vi "set_lc_end.vi"(8 "yw":string, 9 "state":string, 11 "lc_num":string) -> (2 "error":errorcluster)   [LabVIEW 2017, in "Lib_code.lvlib"]
uses:
  Lib_code.lvlib
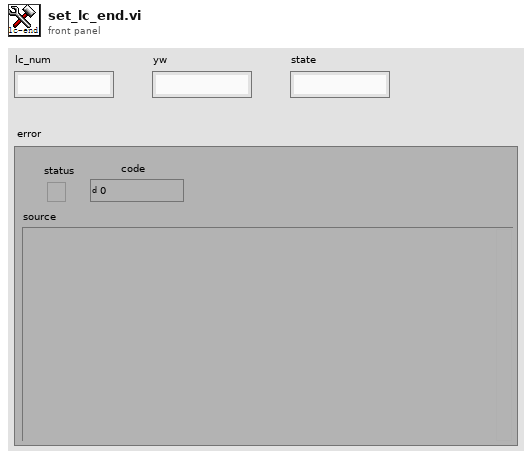
[diagram p1: front panel]
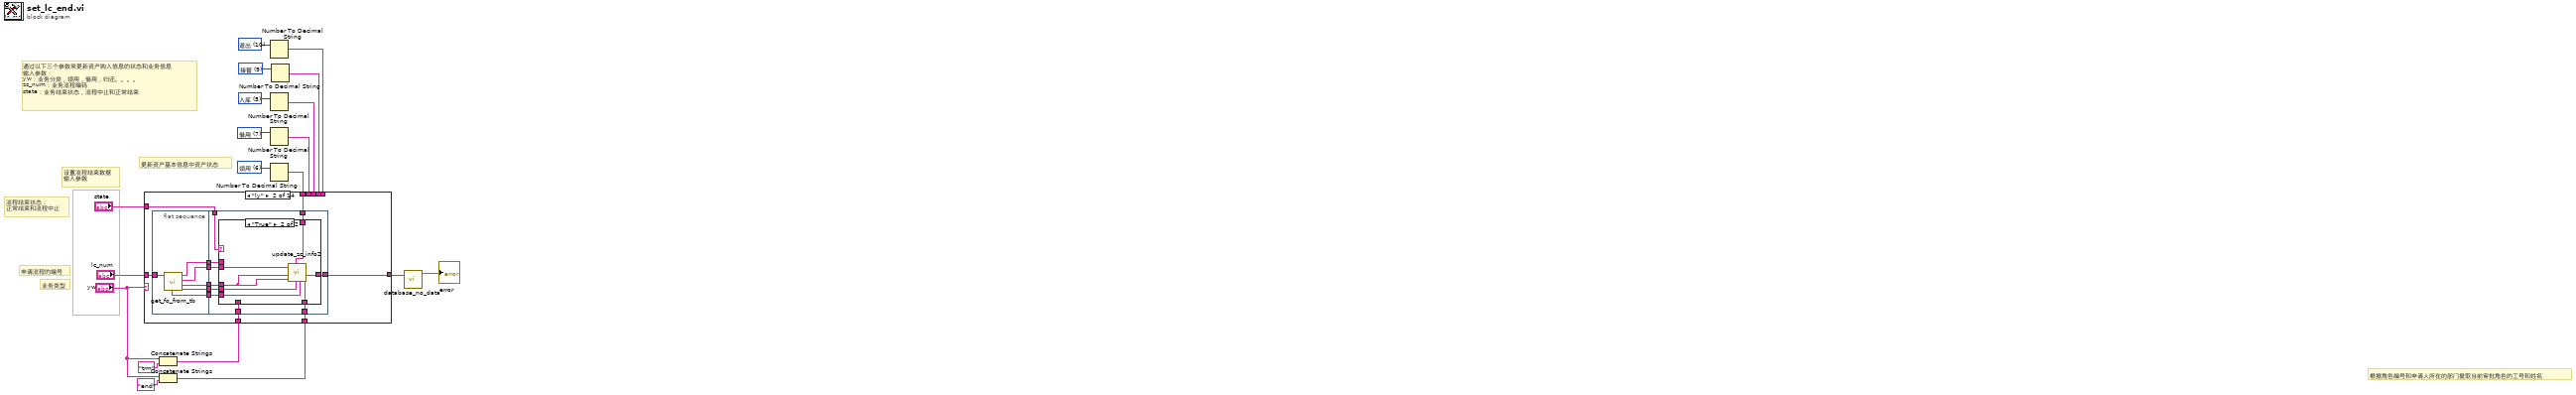
[diagram p0: block diagram]
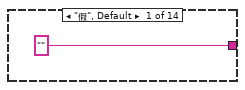
[diagram p2: hidden frame]
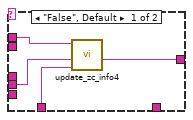
[diagram p3: hidden frame]
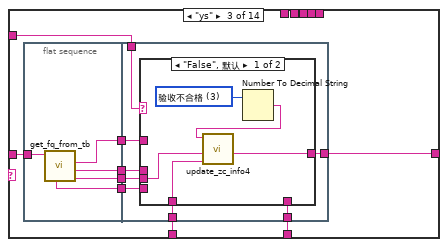
[diagram p4: hidden frame]
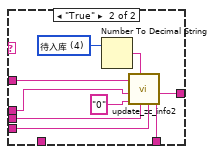
[diagram p5: hidden frame]
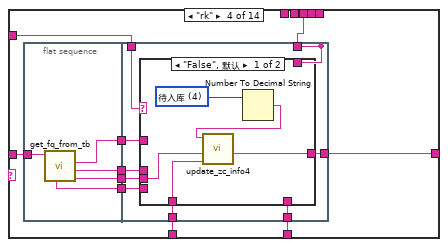
[diagram p6: hidden frame]
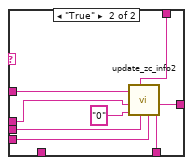
[diagram p7: hidden frame]
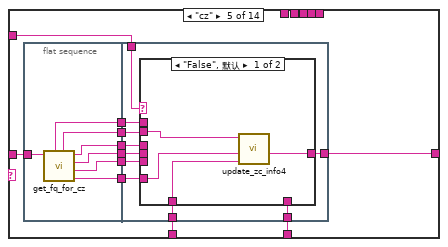
[diagram p8: hidden frame]
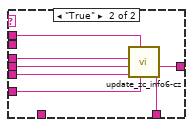
[diagram p9: hidden frame]
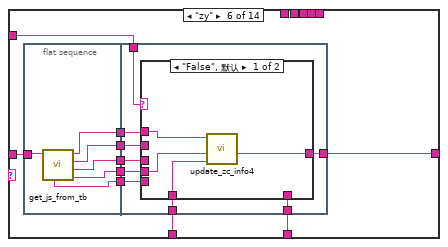
[diagram p10: hidden frame]
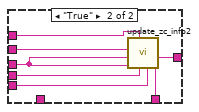
[diagram p11: hidden frame]
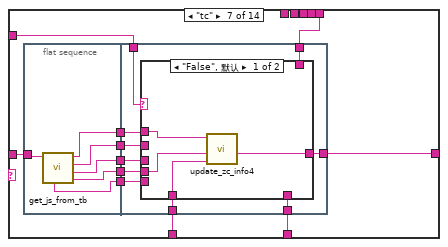
[diagram p12: hidden frame]
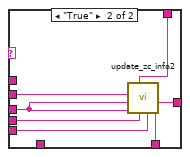
[diagram p13: hidden frame]
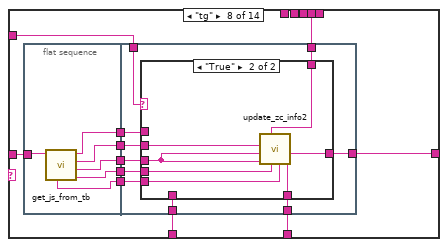
[diagram p14: hidden frame]
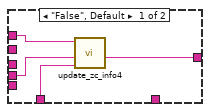
[diagram p15: hidden frame]
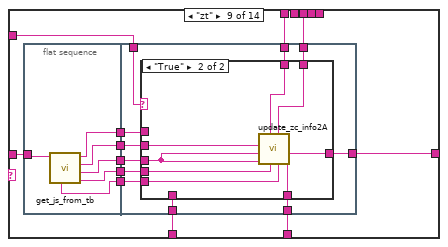
[diagram p16: hidden frame]
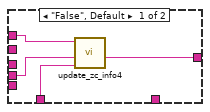
[diagram p17: hidden frame]
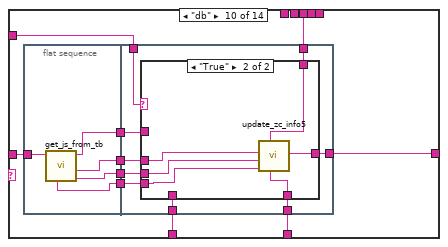
[diagram p18: hidden frame]
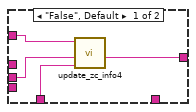
[diagram p19: hidden frame]
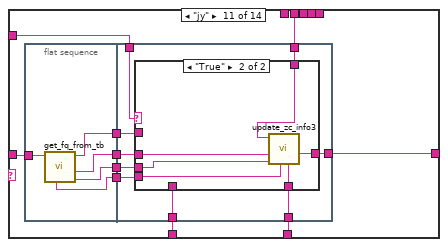
[diagram p20: hidden frame]
diagram:
  w2 = u8 10 items=["待验收"=1, "无需验收"=2, "验收不合格"=3, "待入库"=4, "入库"=5, "领用"=6, "借用"=7, "托管"=8, "接管"=9, "退出"=10, "出库在用"=11, "盘亏"=12, "出售"=13, "报废"=14, "领用中"=120, "退库中"=121, "借用中"=122, "归还中"=123, "转移中"=124, "调拨中"=125, "借调中"=126, "托管中"=127, "终止托管中"=128, "退出中"=129, "处置中"=130] ("借用状态")
  w5 = u8 6 items=["待验收"=1, "无需验收"=2, "验收不合格"=3, "待入库"=4, "入库"=5, "领用"=6, "借用"=7, "托管"=8, "接管"=9, "退出"=10, "出库在用"=11, "盘亏"=12, "出售"=13, "报废"=14, "领用中"=120, "退库中"=121, "借用中"=122, "归还中"=123, "转移中"=124, "调拨中"=125, "借调中"=126, "托管中"=127, "终止托管中"=128, "退出中"=129, "处置中"=130] ("借用状态")
  w6 = u8 7 items=["待验收"=1, "无需验收"=2, "验收不合格"=3, "待入库"=4, "入库"=5, "领用"=6, "借用"=7, "托管"=8, "接管"=9, "退出"=10, "出库在用"=11, "盘亏"=12, "出售"=13, "报废"=14, "领用中"=120, "退库中"=121, "借用中"=122, "归还中"=123, "转移中"=124, "调拨中"=125, "借调中"=126, "托管中"=127, "终止托管中"=128, "退出中"=129, "处置中"=130] ("借用状态")
  w7 = u8 5 items=["待验收"=1, "无需验收"=2, "验收不合格"=3, "待入库"=4, "入库"=5, "领用"=6, "借用"=7, "托管"=8, "接管"=9, "退出"=10, "出库在用"=11, "盘亏"=12, "出售"=13, "报废"=14, "领用中"=120, "退库中"=121, "借用中"=122, "归还中"=123, "转移中"=124, "调拨中"=125, "借调中"=126, "托管中"=127, "终止托管中"=128, "退出中"=129, "处置中"=130] ("借用状态")
  w4 = u8 9 items=["待验收"=1, "无需验收"=2, "验收不合格"=3, "待入库"=4, "入库"=5, "领用"=6, "借用"=7, "托管"=8, "接管"=9, "退出"=10, "出库在用"=11, "盘亏"=12, "出售"=13, "报废"=14, "领用中"=120, "退库中"=121, "借用中"=122, "归还中"=123, "转移中"=124, "调拨中"=125, "借调中"=126, "托管中"=127, "终止托管中"=128, "退出中"=129, "处置中"=130] ("借用状态")
  # "更新资产基本信息中资产状态"
  # "申请流程的编号"
  # "业务类型"
  # "流程结束状态：\n正常结束和流程中止"
  # "设置流程结束数据\n输入参数"
  # "通过以下三个参数来更新资产购入信息的状态和业务信息\n输入参数：\nyw：业务分类，领用，借用，归还。。。。\nzc_num：业务流程编码\nstate：业务结束状态，流程中止和正常结束"
  # "根据角色编号和申请人所在的部门提取当前审批角色的工号和姓名"
  n1 = Concatenate Strings("yw", "trm" ("字符串")) -> (w11:string)
  n2 = Concatenate Strings("yw", "end" ("字符串")) -> (w14:string)
  n3 = Number To Decimal String(number=w7) -> (decimal integer string=w9:string)  [unwired: 1 in]
  n4 = Number To Decimal String(number=w6) -> (decimal integer string=w8:string)  [unwired: 1 in]
  n5 = Number To Decimal String(number=w5) -> (decimal integer string=w10:string)  [unwired: 1 in]
  n6 = Number To Decimal String(number=w2) -> (decimal integer string=w1:string)  [unwired: 1 in]
  n7 = Number To Decimal String(number=w4) -> (decimal integer string=w3:string)  [unwired: 1 in]
  n8 = case shown="\"ly\"" "yw" {
    tunnel: "lc_num" -> [_ w29 w65 w102 w140 w178 w215 w253 w292 w332 w366 w399 w428 w465]
    tunnel: "state" -> [_ w31 w67 w104 w142 w180 w217 w255 w294 w333 w367 w400 w432 w467]
    tunnel: ["" w25 w62 w99 w136 w174 w211 w249 w288 w328 w362 w395 w427 w464] -> w17
    tunnel: w14 -> [_ w24 w61 w98 w135 w173 w210 w248 w287 w327 w361 w394 w426 w463]
    tunnel: w11 -> [_ w23 w60 w97 w134 w172 w209 w247 w286 w326 w360 w393 w425 w462]
    tunnel: w10 -> [_ w21 _ _ _ _ _ _ w284 _ _ _ w422 _]
    tunnel: w9 -> [_ _ _ w95 _ _ _ _ w283 w324 _ _ w423 w460]
    tunnel: w8 -> [_ _ _ _ _ _ _ _ _ _ w358 _ _ w459]
    tunnel: w3 -> [_ _ _ _ _ _ _ w245 _ _ _ _ _ _]
    tunnel: w1 -> [_ _ _ _ _ _ w207 _ _ _ _ _ _ _]
    frame "假", Default {
    }
    frame "ly" {
      n9 = flat-sequence {
        tunnel: w29 -> [w32]
        tunnel: [w35] -> w30
        tunnel: [w37] -> w28
        tunnel: [w34] -> w27
        tunnel: [w36] -> w26
        tunnel: [w33] -> w22
        tunnel: w31 -> [w47]
        tunnel: w30 -> [w45]
        tunnel: w28 -> [w46]
        tunnel: w27 -> [w44]
        tunnel: w26 -> [w43]
        tunnel: [w42] -> w25
        tunnel: w24 -> [w41]
        tunnel: w23 -> [w40]
        tunnel: w22 -> [w39]
        tunnel: w21 -> [w38]
        frame #0 {
          n10 = call "get_fq_from_tb.vi"("lc_num"=w32) -> ("zc_luodi_num"=w36:string, "fqren"=w34:string, "fqbumen"=w35:string, "zc_ini_state"=w37:string, "didian"=w33:string)  [unwired: 5 in, 1 out]
        }
        frame #1 {
          n11 = case shown="\"True\"" w47 {
            tunnel: w46 -> [w50 _]
            tunnel: w45 -> [_ w58]
            tunnel: w44 -> [_ w52]
            tunnel: w43 -> [w49 w57]
            tunnel: [w51 w56] -> w42
            tunnel: w41 -> [_ w55]
            tunnel: w40 -> [w48 _]
            tunnel: w39 -> [_ w54]
            tunnel: w38 -> [_ w53]
            frame "False", Default {
              n12 = call "update_zc_info4.vi"("ywxinxi"=w48, "number"=w49, "status"=w50) -> ("data_str"=w51:string)  [unwired: 8 in]
            }
            frame "True" {
              n13 = call "update_zc_info2.vi"("ywxinxi"=w55, "didian"=w54, "number"=w57, "status"=w53, "syren"=w52, "zrren"=w52, "zrbumen"=w58) -> ("data_str"=w56:string)  [unwired: 4 in]
            }
          }
        }
      }
    }
    frame "ys" {
      n14 = flat-sequence {
        tunnel: w65 -> [w68]
        tunnel: [w71] -> w66
        tunnel: [w70] -> w64
        tunnel: [w72] -> w63
        tunnel: [w69] -> w59
        tunnel: w67 -> [w80]
        tunnel: w66 -> [w79]
        tunnel: w64 -> [w78]
        tunnel: w63 -> [w77]
        tunnel: [w76] -> w62
        tunnel: w61 -> [w75]
        tunnel: w60 -> [w74]
        tunnel: w59 -> [w73]
        frame #0 {
          n15 = call "get_fq_from_tb.vi"("lc_num"=w68) -> ("zc_luodi_num"=w72:string, "fqren"=w70:string, "fqbumen"=w71:string, "didian"=w69:string)  [unwired: 5 in, 2 out]
        }
        frame #1 {
          n16 = case shown="\"False\", 默认" w80 {
            tunnel: w79 -> [_ w94]
            tunnel: w78 -> [_ w89]
            tunnel: w77 -> [w84 w93]
            tunnel: [w85 w92] -> w76
            tunnel: w75 -> [_ w91]
            tunnel: w74 -> [w83 _]
            tunnel: w73 -> [_ w90]
            frame "False", Default {
              w82 = u8 3 items=["待验收"=1, "无需验收"=2, "验收不合格"=3, "待入库"=4, "入库"=5, "领用"=6, "借用"=7, "托管"=8, "接管"=9, "退出"=10, "出库在用"=11, "盘亏"=12, "出售"=13, "报废"=14, "领用中"=120, "退库中"=121, "借用中"=122, "归还中"=123, "转移中"=124, "调拨中"=125, "借调中"=126, "托管中"=127, "终止托管中"=128, "退出中"=129, "处置中"=130] ("借用状态")
              n17 = Number To Decimal String(number=w82) -> (decimal integer string=w81:string)  [unwired: 1 in]
              n18 = call "update_zc_info4.vi"("ywxinxi"=w83, "number"=w84, "status"=w81) -> ("data_str"=w85:string)  [unwired: 8 in]
            }
            frame "True" {
              w87 = u8 4 items=["待验收"=1, "无需验收"=2, "验收不合格"=3, "待入库"=4, "入库"=5, "领用"=6, "借用"=7, "托管"=8, "接管"=9, "退出"=10, "出库在用"=11, "盘亏"=12, "出售"=13, "报废"=14, "领用中"=120, "退库中"=121, "借用中"=122, "归还中"=123, "转移中"=124, "调拨中"=125, "借调中"=126, "托管中"=127, "终止托管中"=128, "退出中"=129, "处置中"=130] ("借用状态")
              n19 = Number To Decimal String(number=w87) -> (decimal integer string=w86:string)  [unwired: 1 in]
              n20 = call "update_zc_info2.vi"("ywxinxi"=w91, "didian"=w90, "number"=w93, "status"=w86, "syren"="0", "zrren"=w89, "zrbumen"=w94) -> ("data_str"=w92:string)  [unwired: 4 in]
            }
          }
        }
      }
    }
    frame "rk" {
      n21 = flat-sequence {
        tunnel: w102 -> [w105]
        tunnel: [w108] -> w103
        tunnel: [w107] -> w101
        tunnel: [w109] -> w100
        tunnel: [w106] -> w96
        tunnel: w104 -> [w118]
        tunnel: w103 -> [w117]
        tunnel: w101 -> [w116]
        tunnel: w100 -> [w115]
        tunnel: [w114] -> w99
        tunnel: w98 -> [w113]
        tunnel: w97 -> [w112]
        tunnel: w96 -> [w111]
        tunnel: [w110] -> _
        tunnel: w95 -> [w110]
        frame #0 {
          n22 = call "get_fq_from_tb.vi"("lc_num"=w105) -> ("zc_luodi_num"=w109:string, "fqren"=w107:string, "fqbumen"=w108:string, "didian"=w106:string)  [unwired: 5 in, 2 out]
        }
        frame #1 {
          n23 = case shown="\"False\", 默认" w118 {
            tunnel: w117 -> [_ w131]
            tunnel: w116 -> [_ w126]
            tunnel: w115 -> [w122 w130]
            tunnel: [w123 w129] -> w114
            tunnel: w113 -> [_ w128]
            tunnel: w112 -> [w121 _]
            tunnel: w111 -> [_ w127]
            tunnel: w110 -> [_ w124]
            frame "False", Default {
              w120 = u8 4 items=["待验收"=1, "无需验收"=2, "验收不合格"=3, "待入库"=4, "入库"=5, "领用"=6, "借用"=7, "托管"=8, "接管"=9, "退出"=10, "出库在用"=11, "盘亏"=12, "出售"=13, "报废"=14, "领用中"=120, "退库中"=121, "借用中"=122, "归还中"=123, "转移中"=124, "调拨中"=125, "借调中"=126, "托管中"=127, "终止托管中"=128, "退出中"=129, "处置中"=130] ("借用状态")
              n24 = Number To Decimal String(number=w120) -> (decimal integer string=w119:string)  [unwired: 1 in]
              n25 = call "update_zc_info4.vi"("ywxinxi"=w121, "number"=w122, "status"=w119) -> ("data_str"=w123:string)  [unwired: 8 in]
            }
            frame "True" {
              n26 = call "update_zc_info2.vi"("ywxinxi"=w128, "didian"=w127, "number"=w130, "status"=w124, "syren"="0", "zrren"=w126, "zrbumen"=w131) -> ("data_str"=w129:string)  [unwired: 4 in]
            }
          }
        }
      }
    }
    frame "cz" {
      n27 = flat-sequence {
        tunnel: w140 -> [w149]
        tunnel: [w146] -> w141
        tunnel: [w148] -> w139
        tunnel: [w145] -> w138
        tunnel: [w147] -> w137
        tunnel: [w144] -> w133
        tunnel: [w143] -> w132
        tunnel: w142 -> [w159]
        tunnel: w141 -> [w157]
        tunnel: w139 -> [w158]
        tunnel: w138 -> [w156]
        tunnel: w137 -> [w155]
        tunnel: [w154] -> w136
        tunnel: w135 -> [w153]
        tunnel: w134 -> [w152]
        tunnel: w133 -> [w151]
        tunnel: w132 -> [w150]
        frame #0 {
          n28 = call "get_fq_for_cz.vi"("lc_num"=w149) -> ("zc_luodi_num"=w147:string, "syren"=w144:string, "fqren"=w145:string, "fqbumen"=w146:string, "zc_ini_state"=w148:string, "fangshi"=w143:string)  [unwired: 4 in, 1 out]
        }
        frame #1 {
          n29 = case shown="\"False\", 默认" w159 {
            tunnel: w158 -> [w162 _]
            tunnel: w157 -> [_ w168]
            tunnel: w156 -> [_ w167]
            tunnel: w155 -> [w161 w165]
            tunnel: [w163 w170] -> w154
            tunnel: w153 -> [_ w164]
            tunnel: w152 -> [w160 _]
            tunnel: w151 -> [_ w166]
            tunnel: w150 -> [_ w169]
            frame "False", Default {
              n30 = call "update_zc_info4.vi"("ywxinxi"=w160, "number"=w161, "status"=w162) -> ("data_str"=w163:string)  [unwired: 8 in]
            }
            frame "True" {
              n31 = call "update_zc_info6-cz.vi"("ywxinxi"=w164, "number"=w165, "status"=w169, "syren"=w166, "zrren"=w167, "zrbumen"=w168) -> ("data_str"=w170:string)  [unwired: 5 in]
            }
          }
        }
      }
    }
    frame "zy" {
      n32 = flat-sequence {
        tunnel: w178 -> [w186]
        tunnel: [w184] -> w179
        tunnel: [w185] -> w177
        tunnel: [w183] -> w176
        tunnel: [w182] -> w175
        tunnel: [w181] -> w171
        tunnel: w180 -> [w195]
        tunnel: w179 -> [w193]
        tunnel: w177 -> [w194]
        tunnel: w176 -> [w192]
        tunnel: w175 -> [w191]
        tunnel: [w190] -> w174
        tunnel: w173 -> [w189]
        tunnel: w172 -> [w188]
        tunnel: w171 -> [w187]
        frame #0 {
          n33 = call "get_js_from_tb.vi"("lc_num"=w186) -> ("zc_luodi_num"=w182:string, "jsren"=w183:string, "jsbumen"=w184:string, "zc_ini_state"=w185:string, "didian"=w181:string)  [unwired: 5 in, 1 out]
        }
        frame #1 {
          n34 = case shown="\"False\", 默认" w195 {
            tunnel: w194 -> [w199 w200]
            tunnel: w193 -> [_ w205]
            tunnel: w192 -> [_ w204]
            tunnel: w191 -> [w198 w203]
            tunnel: [w196 w206] -> w190
            tunnel: w189 -> [_ w202]
            tunnel: w188 -> [w197 _]
            tunnel: w187 -> [_ w201]
            frame "False", Default {
              n35 = call "update_zc_info4.vi"("ywxinxi"=w197, "number"=w198, "status"=w199) -> ("data_str"=w196:string)  [unwired: 8 in]
            }
            frame "True" {
              n36 = call "update_zc_info2.vi"("ywxinxi"=w202, "didian"=w201, "number"=w203, "status"=w200, "syren"=w204, "zrren"=w204, "zrbumen"=w205) -> ("data_str"=w206:string)  [unwired: 4 in]
            }
          }
        }
      }
    }
    frame "tc" {
      n37 = flat-sequence {
        tunnel: w215 -> [w223]
        tunnel: [w219] -> w216
        tunnel: [w218] -> w214
        tunnel: [w220] -> w213
        tunnel: [w221] -> w212
        tunnel: [w222] -> w208
        tunnel: w217 -> [w233]
        tunnel: w216 -> [w231]
        tunnel: w214 -> [w232]
        tunnel: w213 -> [w230]
        tunnel: w212 -> [w229]
        tunnel: [w228] -> w211
        tunnel: w210 -> [w227]
        tunnel: w209 -> [w226]
        tunnel: w208 -> [w225]
        tunnel: w207 -> [w224]
        frame #0 {
          n38 = call "get_js_from_tb.vi"("lc_num"=w223) -> ("zc_luodi_num"=w221:string, "jsren"=w220:string, "jsbumen"=w219:string, "zc_ini_state"=w218:string, "didian"=w222:string)  [unwired: 5 in, 1 out]
        }
        frame #1 {
          n39 = case shown="\"False\", 默认" w233 {
            tunnel: w232 -> [w237 _]
            tunnel: w231 -> [_ w243]
            tunnel: w230 -> [_ w242]
            tunnel: w229 -> [w236 w241]
            tunnel: [w234 w244] -> w228
            tunnel: w227 -> [_ w240]
            tunnel: w226 -> [w235 _]
            tunnel: w225 -> [_ w239]
            tunnel: w224 -> [_ w238]
            frame "False", Default {
              n40 = call "update_zc_info4.vi"("ywxinxi"=w235, "number"=w236, "status"=w237) -> ("data_str"=w234:string)  [unwired: 8 in]
            }
            frame "True" {
              n41 = call "update_zc_info2.vi"("ywxinxi"=w240, "didian"=w239, "number"=w241, "status"=w238, "syren"=w242, "zrren"=w242, "zrbumen"=w243) -> ("data_str"=w244:string)  [unwired: 4 in]
            }
          }
        }
      }
    }
    frame "tg" {
      n42 = flat-sequence {
        tunnel: w253 -> [w261]
        tunnel: [w257] -> w254
        tunnel: [w256] -> w252
        tunnel: [w258] -> w251
        tunnel: [w259] -> w250
        tunnel: [w260] -> w246
        tunnel: w255 -> [w271]
        tunnel: w254 -> [w269]
        tunnel: w252 -> [w270]
        tunnel: w251 -> [w268]
        tunnel: w250 -> [w267]
        tunnel: [w266] -> w249
        tunnel: w248 -> [w265]
        tunnel: w247 -> [w264]
        tunnel: w246 -> [w263]
        tunnel: w245 -> [w262]
        frame #0 {
          n43 = call "get_js_from_tb.vi"("lc_num"=w261) -> ("zc_luodi_num"=w259:string, "jsren"=w258:string, "jsbumen"=w257:string, "zc_ini_state"=w256:string, "didian"=w260:string)  [unwired: 5 in, 1 out]
        }
        frame #1 {
          n44 = case shown="\"True\"" w271 {
            tunnel: w270 -> [w275 _]
            tunnel: w269 -> [_ w281]
            tunnel: w268 -> [_ w280]
            tunnel: w267 -> [w274 w279]
            tunnel: [w272 w282] -> w266
            tunnel: w265 -> [_ w278]
            tunnel: w264 -> [w273 _]
            tunnel: w263 -> [_ w277]
            tunnel: w262 -> [_ w276]
            frame "False", Default {
              n45 = call "update_zc_info4.vi"("ywxinxi"=w273, "number"=w274, "status"=w275) -> ("data_str"=w272:string)  [unwired: 8 in]
            }
            frame "True" {
              n46 = call "update_zc_info2.vi"("ywxinxi"=w278, "didian"=w277, "number"=w279, "status"=w276, "syren"=w280, "zrren"=w280, "zrbumen"=w281) -> ("data_str"=w282:string)  [unwired: 4 in]
            }
          }
        }
      }
    }
    frame "zt" {
      n47 = flat-sequence {
        tunnel: w292 -> [w300]
        tunnel: [w296] -> w293
        tunnel: [w295] -> w291
        tunnel: [w297] -> w290
        tunnel: [w298] -> w289
        tunnel: [w299] -> w285
        tunnel: w294 -> [w311]
        tunnel: w293 -> [w309]
        tunnel: w291 -> [w310]
        tunnel: w290 -> [w308]
        tunnel: w289 -> [w307]
        tunnel: [w306] -> w288
        tunnel: w287 -> [w305]
        tunnel: w286 -> [w304]
        tunnel: w285 -> [w303]
        tunnel: w284 -> [w302]
        tunnel: w283 -> [w301]
        frame #0 {
          n48 = call "get_js_from_tb.vi"("lc_num"=w300) -> ("zc_luodi_num"=w298:string, "jsren"=w297:string, "jsbumen"=w296:string, "zc_ini_state"=w295:string, "didian"=w299:string)  [unwired: 5 in, 1 out]
        }
        frame #1 {
          n49 = case shown="\"True\"" w311 {
            tunnel: w310 -> [w315 _]
            tunnel: w309 -> [_ w322]
            tunnel: w308 -> [_ w321]
            tunnel: w307 -> [w314 w320]
            tunnel: [w312 w323] -> w306
            tunnel: w305 -> [_ w318]
            tunnel: w304 -> [w313 _]
            tunnel: w303 -> [_ w319]
            tunnel: w302 -> [_ w317]
            tunnel: w301 -> [_ w316]
            frame "False", Default {
              n50 = call "update_zc_info4.vi"("ywxinxi"=w313, "number"=w314, "status"=w315) -> ("data_str"=w312:string)  [unwired: 8 in]
            }
            frame "True" {
              n51 = call "update_zc_info2A.vi"("ywxinxi"=w318, "didian"=w319, "ruku"=w316, "number"=w320, "lingyong"=w317, "syren"=w321, "zrren"=w321, "zrbumen"=w322) -> ("data_str"=w323:string)  [unwired: 3 in]
            }
          }
        }
      }
    }
    frame "db" {
      n52 = flat-sequence {
        tunnel: w332 -> [w338]
        tunnel: [w334] -> w331
        tunnel: [w335] -> w330
        tunnel: [w336] -> w329
        tunnel: [w337] -> w325
        tunnel: w333 -> [w347]
        tunnel: w331 -> [w346]
        tunnel: w330 -> [w345]
        tunnel: w329 -> [w344]
        tunnel: [w343] -> w328
        tunnel: w327 -> [w342]
        tunnel: w326 -> [w341]
        tunnel: w325 -> [w340]
        tunnel: w324 -> [w339]
        frame #0 {
          n53 = call "get_js_from_tb.vi"("lc_num"=w338) -> ("zc_luodi_num"=w336:string, "jsren"=w335:string, "zc_ini_state"=w334:string, "didian"=w337:string)  [unwired: 5 in, 2 out]
        }
        frame #1 {
          n54 = case shown="\"True\"" w347 {
            tunnel: w346 -> [w351 _]
            tunnel: w345 -> [_ w356]
            tunnel: w344 -> [w350 w355]
            tunnel: [w348 w357] -> w343
            tunnel: w342 -> [_ w354]
            tunnel: w341 -> [w349 _]
            tunnel: w340 -> [_ w353]
            tunnel: w339 -> [_ w352]
            frame "False", Default {
              n55 = call "update_zc_info4.vi"("ywxinxi"=w349, "number"=w350, "status"=w351) -> ("data_str"=w348:string)  [unwired: 8 in]
            }
            frame "True" {
              n56 = call "update_zc_info5.vi"("ywxinxi"=w354, "status"=w352, "didian"=w353, "number"=w355, "zerenren"=w356) -> ("data_str"=w357:string)  [unwired: 6 in]
            }
          }
        }
      }
    }
    frame "jy" {
      n57 = flat-sequence {
        tunnel: w366 -> [w368]
        tunnel: [w370] -> w365
        tunnel: [w371] -> w364
        tunnel: [w372] -> w363
        tunnel: [w369] -> w359
        tunnel: w367 -> [w381]
        tunnel: w365 -> [w380]
        tunnel: w364 -> [w379]
        tunnel: w363 -> [w378]
        tunnel: [w377] -> w362
        tunnel: w361 -> [w376]
        tunnel: w360 -> [w375]
        tunnel: w359 -> [w374]
        tunnel: w358 -> [w373]
        frame #0 {
          n58 = call "get_fq_from_tb.vi"("lc_num"=w368) -> ("zc_luodi_num"=w372:string, "fqren"=w371:string, "zc_ini_state"=w370:string, "didian"=w369:string)  [unwired: 5 in, 2 out]
        }
        frame #1 {
          n59 = case shown="\"True\"" w381 {
            tunnel: w380 -> [w384 _]
            tunnel: w379 -> [_ w390]
            tunnel: w378 -> [w383 w389]
            tunnel: [w385 w391] -> w377
            tunnel: w376 -> [_ w388]
            tunnel: w375 -> [w382 _]
            tunnel: w374 -> [_ w387]
            tunnel: w373 -> [_ w386]
            frame "False", Default {
              n60 = call "update_zc_info4.vi"("ywxinxi"=w382, "number"=w383, "status"=w384) -> ("data_str"=w385:string)  [unwired: 8 in]
            }
            frame "True" {
              n61 = call "update_zc_info3.vi"("ywxinxi"=w388, "didian"=w387, "number"=w389, "syren"=w390, "status"=w386) -> ("data_str"=w391:string)  [unwired: 6 in]
            }
          }
        }
      }
    }
    frame "jd" {
      n62 = flat-sequence {
        tunnel: w399 -> [w401]
        tunnel: [w403] -> w398
        tunnel: [w404] -> w397
        tunnel: [w405] -> w396
        tunnel: [w402] -> w392
        tunnel: w400 -> [w413]
        tunnel: w398 -> [w412]
        tunnel: w397 -> [w411]
        tunnel: w396 -> [w410]
        tunnel: [w409] -> w395
        tunnel: w394 -> [w408]
        tunnel: w393 -> [w407]
        tunnel: w392 -> [w406]
        frame #0 {
          n63 = call "get_fq_from_tb.vi"("lc_num"=w401) -> ("zc_luodi_num"=w405:string, "fqren"=w404:string, "zc_ini_state"=w403:string, "didian"=w402:string)  [unwired: 5 in, 2 out]
        }
        frame #1 {
          n64 = case shown="\"False\", 默认" w413 {
            tunnel: w412 -> [w416 w418]
            tunnel: w411 -> [_ _]
            tunnel: w410 -> [w415 w420]
            tunnel: [w417 w421] -> w409
            tunnel: w408 -> [_ w419]
            tunnel: w407 -> [w414 _]
            tunnel: w406 -> [_ _]
            frame "False", Default {
              n65 = call "update_zc_info4.vi"("ywxinxi"=w414, "number"=w415, "status"=w416) -> ("data_str"=w417:string)  [unwired: 8 in]
            }
            frame "True" {
              n66 = call "update_zc_info4.vi"("ywxinxi"=w419, "number"=w420, "status"=w418) -> ("data_str"=w421:string)  [unwired: 8 in]
            }
          }
        }
      }
    }
    frame "tk" {
      n67 = flat-sequence {
        tunnel: [w435] -> w431
        tunnel: [w433] -> w430
        tunnel: [w434] -> w429
        tunnel: w428 -> [w437]
        tunnel: [w436] -> w424
        tunnel: w432 -> [w447]
        tunnel: w431 -> [w446]
        tunnel: w430 -> [w445]
        tunnel: w429 -> [w444]
        tunnel: [w443] -> w427
        tunnel: w426 -> [w442]
        tunnel: w425 -> [w441]
        tunnel: w424 -> [w440]
        tunnel: w423 -> [w439]
        tunnel: w422 -> [w438]
        frame #0 {
          n68 = call "get_js_from_tb2.vi"("lc_num"=w437) -> ("zc_luodi_num"=w435:string, "jsren"=w434:string, "jsbumen"=w433:string, "didian"=w436:string)  [unwired: 6 in, 1 out]
        }
        frame #1 {
          n69 = case shown="\"True\"" w447 {
            tunnel: w445 -> [_ w457]
            tunnel: w444 -> [_ w455]
            tunnel: w446 -> [w450 w456]
            tunnel: [w451 w458] -> w443
            tunnel: w442 -> [_ w454]
            tunnel: w441 -> [w449 _]
            tunnel: w440 -> [_ w453]
            tunnel: w439 -> [_ w452]
            tunnel: w438 -> [w448 _]
            frame "False", Default {
              n70 = call "update_zc_info4.vi"("ywxinxi"=w449, "number"=w450, "status"=w448) -> ("data_str"=w451:string)  [unwired: 8 in]
            }
            frame "True" {
              n71 = call "update_zc_info2.vi"("ywxinxi"=w454, "didian"=w453, "number"=w456, "status"=w452, "syren"=w455, "zrren"=w455, "zrbumen"=w457) -> ("data_str"=w458:string)  [unwired: 4 in]
            }
          }
        }
      }
    }
    frame "gh" {
      n72 = flat-sequence {
        tunnel: [w468] -> w466
        tunnel: w465 -> [w470]
        tunnel: [w469] -> w461
        tunnel: w467 -> [w478]
        tunnel: w466 -> [w477]
        tunnel: [w476] -> w464
        tunnel: w463 -> [w475]
        tunnel: w462 -> [w474]
        tunnel: w461 -> [w473]
        tunnel: w460 -> [w472]
        tunnel: w459 -> [w471]
        frame #0 {
          n73 = call "get_js_from_tb2.vi"("lc_num"=w470) -> ("zc_luodi_num"=w468:string, "didian"=w469:string)  [unwired: 6 in, 3 out]
        }
        frame #1 {
          n74 = case shown="\"True\"" w478 {
            tunnel: w477 -> [w481 w487]
            tunnel: [w482 w488] -> w476
            tunnel: w475 -> [_ w486]
            tunnel: w474 -> [w480 _]
            tunnel: w473 -> [_ w485]
            tunnel: w472 -> [_ w484]
            tunnel: w471 -> [w479 _]
            frame "False", Default {
              n75 = call "update_zc_info4.vi"("ywxinxi"=w480, "number"=w481, "status"=w479) -> ("data_str"=w482:string)  [unwired: 8 in]
            }
            frame "True" {
              n76 = call "update_zc_info3.vi"("ywxinxi"=w486, "didian"=w485, "number"=w487, "syren"="0", "status"=w484) -> ("data_str"=w488:string)  [unwired: 6 in]
            }
          }
        }
      }
    }
  }
  n77 = call "database_no_data.vi"("input"=w17) -> ("error"=→"error":errorcluster)  [unwired: 2 in]
